vi "Write Flow Control.vi"(8 "error in (no error)":errorcluster, 10 "Flow Control":u16(ring) items=["None", "XON/XOFF", "RTS/CTS", "XON/XOFF & RTS/CTS", "DTR/DSR", "XON/XOFF & DTR/DSR"], 11 "Serial Master in":refnum<class "Serial Master.lvclass">) -> (0 "error out":errorcluster, 3 "Serial Master out":refnum<class "Serial Master.lvclass">)   [LabVIEW 2013, in "Modbus Library - Advance.lvlib" / "Serial Master.lvclass"]
uses:
  Serial Master.lvclass
  Serial Master.lvclass/Serial Master.ctl
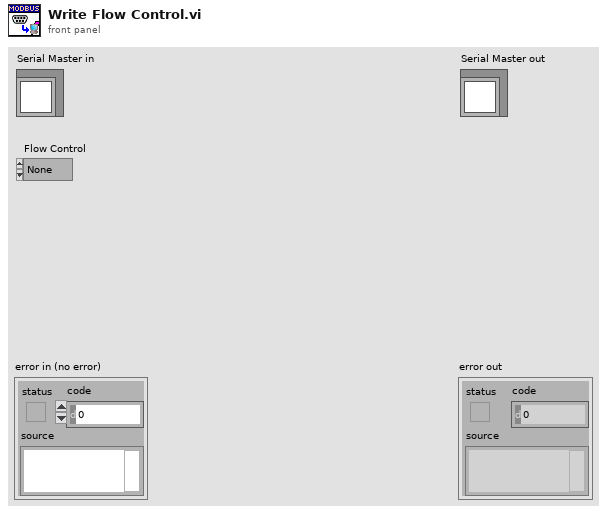
[diagram p1: front panel]
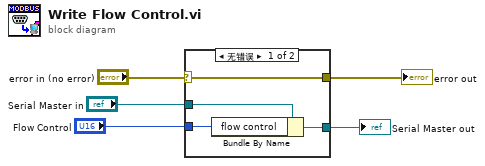
[diagram p0: block diagram]
diagram:
  n1 = case shown="无错误" "error in (no error)" {
    selector: "error in (no error)" -> [w9 w10]
    tunnel: [w9 w10] -> w4
    tunnel: [w7 w11] -> w2
    tunnel: "Serial Master in" -> [w8 w11]
    tunnel: "Flow Control" -> [w6 _]
    frame No Error {
      n2 = Bundle By Name(cluster=w8, "flow control"=w6) -> (w7:refnum<class "Serial Master.lvclass">)
    }
    frame Error {
    }
  }
  "error out" <- w4
  "Serial Master out" <- w2
